vi "Emballage_BDD_GPAO_V_ARTICLE_ID_ARTICLE.vi"(0 "ID_ARTICLE":string, 11 "error in (no error)":errorcluster) -> (4 "Donnee_header":string[][](array[string]), 6 "Colonne":string[](array[string])=["NOS_ARTICLE", "SUFFIXE", "CLC_DESIGNATION", "INDICE_REV", "ENR_ANNULE", "NB_PIECE_EMB", "REVIS_SUFF"], 8 "Donnée":string[](array[string]), 10 "Enr_Annule":bool, 15 "error out":errorcluster)   [LabVIEW 2020]
uses:
  Modules/FS/60_FS_Controles/60_FS_SetGet.ctl
  <vilib>/addons/database/Connection.llb/DB Tools Open Connec (Path).vi
  <vilib>/addons/database/Connection.llb/Conn Execute.vi
  <vilib>/addons/database/Recordset.llb/Rec Fetch Recordset Data (R).vi
  <vilib>/addons/database/Recordset.llb/Rec Destroy - Connection.vi
  <vilib>/addons/database/NI_Database_API.lvlib
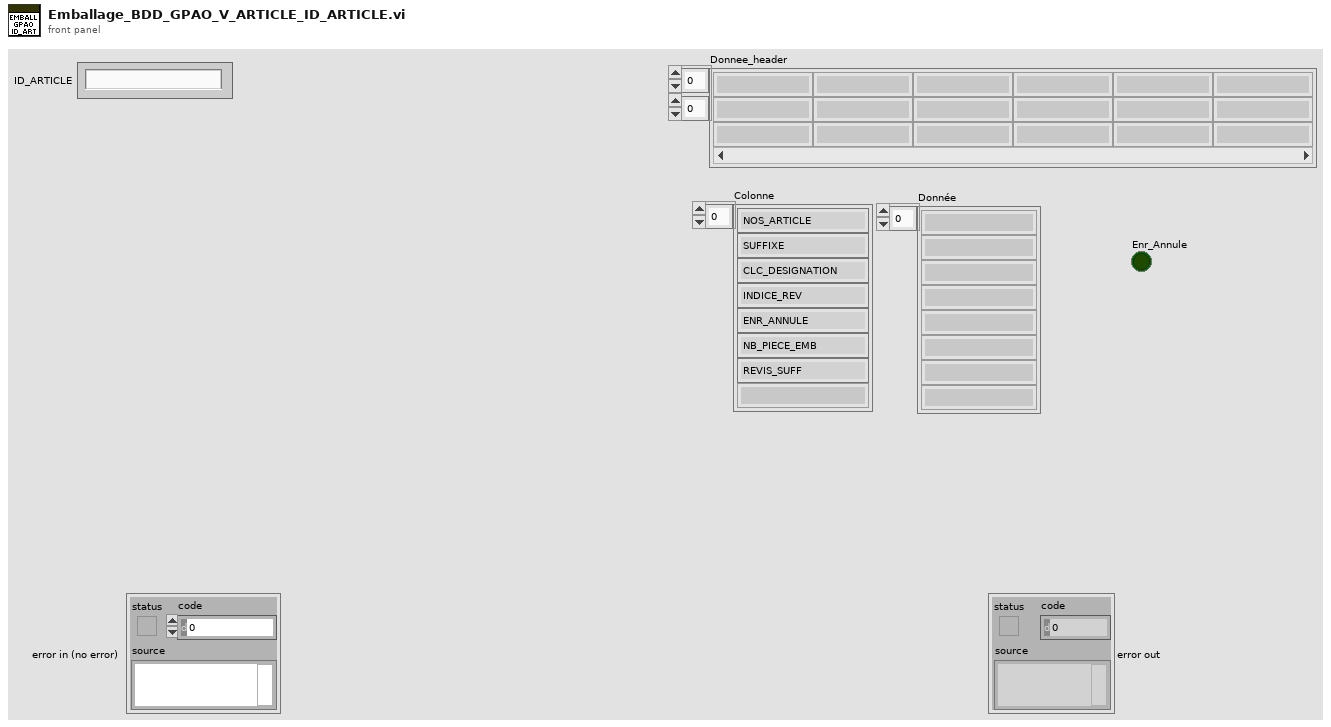
[diagram p1: front panel]
types:
  T1 = typedef "60_FS_SetGet.ctl" = enum16{"set", "get"}
  T2 = typedef "60_FS_CLT_Chemins.ctl" = cluster{"Racine_local":path, "Racine_reseau":path, "Racine_Support_Application":path, "Fichier_Journalisation":path, "Connexion_BDD_VSX":path, "Connexion_BDD_PLZ":path}
  T3 = typedef "NI_Database_API.lvlib/Conn ObjectReference.ctl" = refnum<k1>
  T4 = typedef "NI_Database_API.lvlib/Rec ObjectReference.ctl" = refnum<k1>
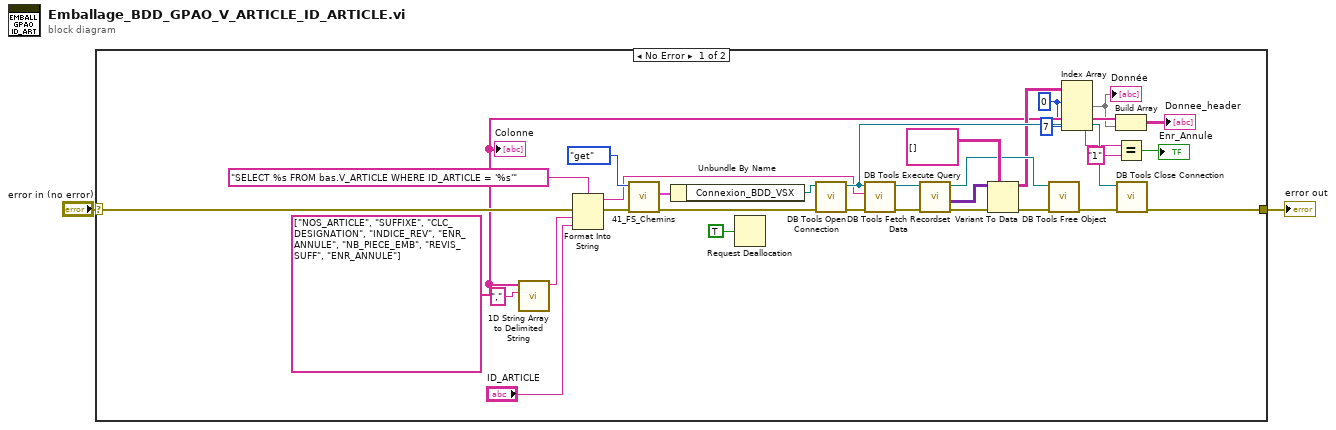
[diagram p0: block diagram]
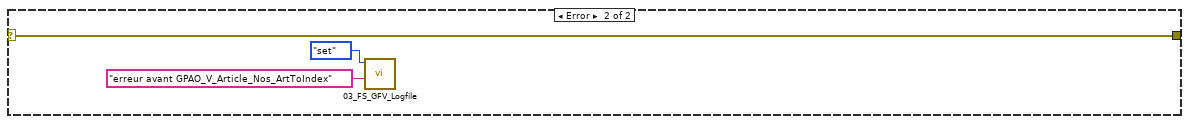
[diagram p2: hidden frame]
diagram:
  n1 = case shown="No Error" "error in (no error)" {
    selector: "error in (no error)" -> [w12 w37]
    tunnel: [w19 w37] -> w1
    frame No Error {
      w10 = string[] ["NOS_ARTICLE", "SUFFIXE", "CLC_DESIGNATION", "INDICE_REV", "ENR_ANNULE", "NB_PIECE_EMB", "REVIS_SUFF", "ENR_ANNULE"]
      w7 = 0 ("indice (ligne)")
      n2 = call <vilib>:"1D String Array to Delimited String.vi"("delimiter"=",", "string array"=w10) -> ("delimited string"=w13:string)  [unwired: 9 in]
      n3 = Format Into String(format string="SELECT %s FROM bas.V_ARTICLE WHERE ID_ARTICLE = '%s'" ("Requète"), error in=w12, w13, "ID_ARTICLE") -> (resulting string=w17:string, error out=w11:errorcluster)  [unwired: 1 in]
      n4 = call "41_FS_Chemins.vi"("error in (no error)"=w11, "SetGet"=60_FS_SetGet."get") -> ("error out"=w32:errorcluster, "CLT_Chemins_out"=w33:T2)  [unwired: 8 in]
      n5 = Unbundle By Name(w33) -> ("Connexion_BDD_VSX"=w23:path)
      n6 = Request Deallocation(TRUE ("flag")) -> ()
      n7 = call-poly <vilib>:"DB Tools Open Connection.vi"("error in (no error)"=w32, "connection information"=w23) -> ("error out"=w21:errorcluster, "connection reference"=w22:T3)  [unwired: 6 in]
      n8 = call-poly <vilib>:"DB Tools Execute Query.vi"("error in (no error)"=w21, "SQL query"=w17, "connection reference"=w22) -> ("error out"=w31:errorcluster, "recordset reference"=w30:T4)  [unwired: 5 in]
      n9 = call-poly <vilib>:"DB Tools Fetch Recordset Data.vi"("error in (no error)"=w31, "recordset reference"=w30) -> ("error out"=w27:errorcluster, "recordset data"=w28:variant[][], "recordset reference out"=w25:T4)  [unwired: 3 in]
      n10 = Variant To Data(error in=w27, type=string[][] [] ("Chaînes []"), Variant=w28) -> (data=w15:string[][], error out=w26:errorcluster)
      n11 = call-poly <vilib>:"DB Tools Free Object.vi"("error in (no error)"=w26, "recordset reference"=w25) -> ("error out"=w24:errorcluster)  [unwired: 8 in, 1 out]
      n12 = Index Array(array=w15, index (row) #1=w7, index (row) #2=w7, index (col) #2=7 ("disabled index (col)")) -> (element #1=w9:string[], element #2=w5:string)  [unwired: 1 in]
      "Donnée" <- w9
      n13 = Build Array(w10, w9) -> (→"Donnee_header":string[][])
      n14 = Equal?(x=w5, y="1") -> (x = y?=→"Enr_Annule":bool)
      n15 = call <vilib>:"DB Tools Close Connection.vi"("error in (no error)"=w24, "connection reference"=w22) -> ("error out"=w19:errorcluster)  [unwired: 5 in]
      "Colonne" <- w10
    }
    frame Error {
      n16 = call "03_FS_GFV_Logfile.vi"("Chaîne"="erreur avant GPAO_V_Article_Nos_ArtToIndex", "States"=60_FS_SetGet."set") -> ()  [unwired: 8 in, 2 out]
    }
  }
  "error out" <- w1
